vi "Write cluster of jsons.vi"(8 "error in (no error)":errorcluster, 10 "cluster of jsons":T1, 11 "Save Image in":refnum<class "Save SPARC4 image.lvclass">) -> (0 "error out":errorcluster, 3 "Save Image out":refnum<class "Save SPARC4 image.lvclass">)   [LabVIEW 2018, in "Save SPARC4 image.lvclass"]
uses:
  Save SPARC4 image.lvclass
  Save SPARC4 image.lvclass/Save SPARC4 image.ctl
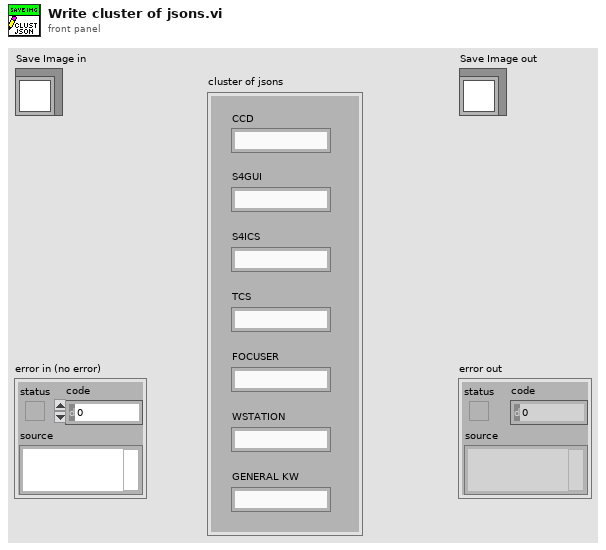
[diagram p1: front panel]
types:
  T1 = cluster{"CCD":string, "S4GUI":string, "S4ICS":string, "TCS":string, "FOCUSER":string, "WSTATION":string, "GENERAL KW":string}
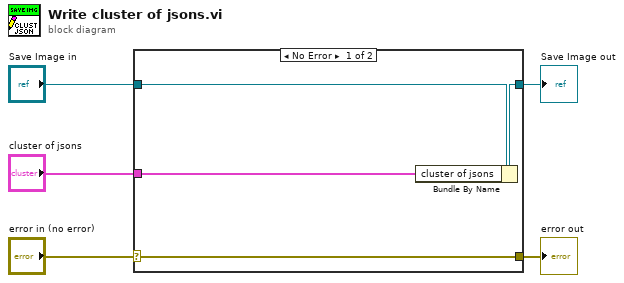
[diagram p0: block diagram]
diagram:
  n1 = case shown="No Error" "error in (no error)" {
    selector: "error in (no error)" -> [w9 w10]
    tunnel: [w9 w10] -> w4
    tunnel: [w7 w11] -> w2
    tunnel: "Save Image in" -> [w8 w11]
    tunnel: "cluster of jsons" -> [w6 _]
    frame No Error {
      n2 = Bundle By Name(cluster=w8, "cluster of jsons"=w6) -> (w7:refnum<class "Save SPARC4 image.lvclass">)
    }
    frame Error {
    }
  }
  "error out" <- w4
  "Save Image out" <- w2
